vi "Get CIPC Reference.vi"(8 "error in (no error)":errorcluster, 10 "Channel Index":i32, 11 "CIFCorePlugin in":refnum<class "CIFCorePlugin.lvclass">) -> (0 "error out":errorcluster, 2 "CIPC Channel":u64, 3 "CIFCorePlugin out":refnum<class "CIFCorePlugin.lvclass">)   [LabVIEW 2021, in "CIFCorePlugin.lvclass"]
doc: "This advanced API provides the direct CIPC reference for channels (assuming CIPC is used by the channel)."
uses:
  CIFCorePlugin.lvclass
  CIFCorePlugin.lvclass/CIFCorePlugin.ctl
  <vilib>/CIF Foundation/CIF Channels Core/CIFChannels/CIFChannels.lvclass
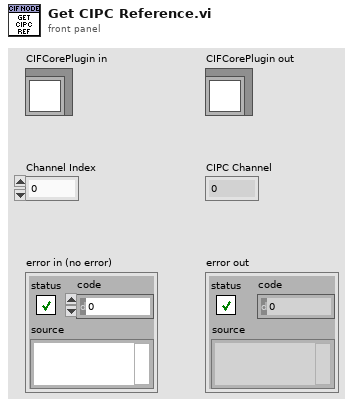
[diagram p1: front panel]
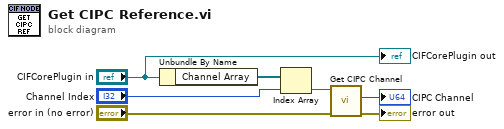
[diagram p0: block diagram]
diagram:
  n1 = Unbundle By Name("CIFCorePlugin in") -> ("Channel Array"=w3:refnum<class "CIFChannels.lvclass">[])
  n2 = Index Array(array=w3, index="Channel Index") -> (element=w2:refnum<class "CIFChannels.lvclass">)
  n3 = call-dynamic "Get CIPC Channel.vi"("error in (no error)"="error in (no error)", "CIFChannels in"=w2) -> ("error out"=→"error out":errorcluster, "CIPC Channel"=→"CIPC Channel":u64)  [unwired: 7 in, 1 out]
  "CIFCorePlugin out" <- "CIFCorePlugin in"
